vi "Tag Watchlist Example.vi"() -> ()   [LabVIEW 2020]
uses:
  Tag/Tag.lvclass/Tag.ctl
  e068aabd-e1ea-42e0-beff-873828abce71.vi
  d3806a0d-e09d-4e85-9d5e-98b09324ad8a.vi
  Tag/Construct.vi
  Core/Write Tag Value_ByRef.vi
  Tag/Write Value with Timestamp.vi
  Tag/Set Properties from Initial.vi
  Core/Add Tag.vi
  Tag/Tag.lvclass
  Core/Tag Core.lvclass
  Watchlist/Tag Watchlist.lvlib
  26ea3595-a312-4975-b521-b090e0f49d92.vi
panel:
  in  "Launch Watchlist":bool
  in  "stop":bool
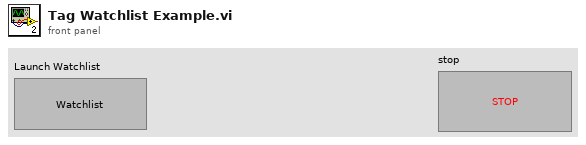
[diagram p1: front panel]
types:
  T1 = cluster{"Name":string, "Value":dbl, "Enable":bool}
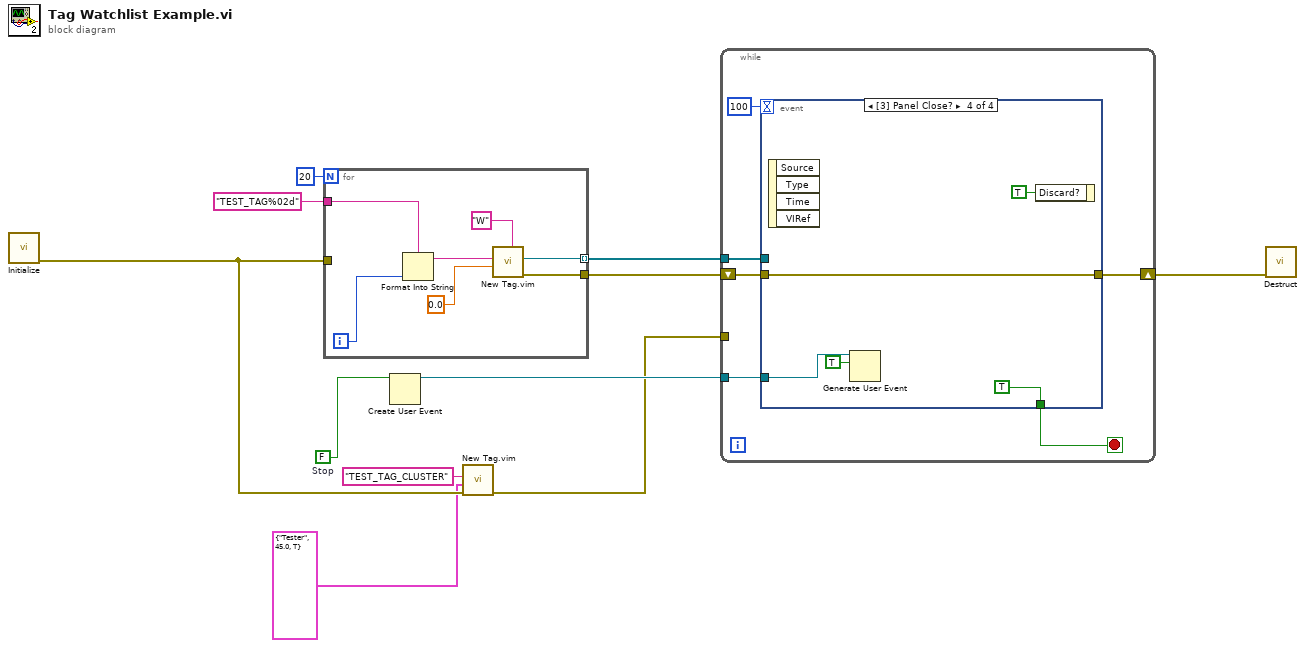
[diagram p0: block diagram]
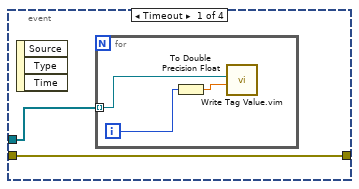
[diagram p2: hidden frame]
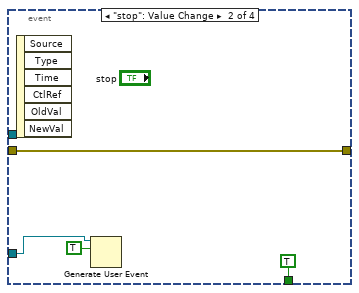
[diagram p3: hidden frame]
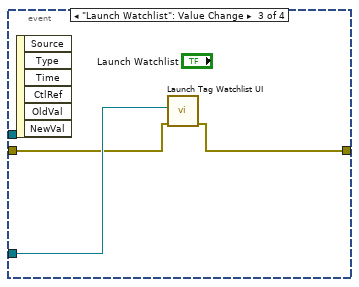
[diagram p4: hidden frame]
diagram:
  w7 = FALSE  # Stop
  n1 = call "Initialize.vi"() -> ("error out"=w4:errorcluster)  [unwired: 11 in]
  n2 = for {
    N: 20 -> [_]
    tunnel: "TEST_TAG%02d" -> [w18]
    tunnel: [w14] -> w9
    tunnel: [w13] -> w5 mode=indexing
    tunnel: w4 -> [_]
    i -> [w17]
    n3 = Format Into String(format string=w18, w17) -> (resulting string=w16:string)  [unwired: 2 in, 1 out]
    n4 = call "New Tag.vim"("Units (none)"="W", "Initial Value"=0.0, "Tag Name"=w16) -> ("error out"=w14:errorcluster, "Tag Ref out"=w13:refnum<data-value>)  [unwired: 7 in]
  }
  n5 = Create User Event(user event datatype=w7) -> (user event=w6:refnum<user-event>)  [unwired: 1 in, 1 out]
  n6 = call "New Tag.vim"("error in (no error)"=w4, "Initial Value"=T1 {"Name"="Tester", "Value"=45.0, "Enable"=TRUE}, "Tag Name"="TEST_TAG_CLUSTER") -> ("error out"=w1:errorcluster)  [unwired: 7 in, 1 out]
  n7 = while {
    shift-right: [w22] -> w8
    shift-left: w9 -> [w23]
    tunnel: w6 -> [w21]
    tunnel: w5 -> [w19]
    tunnel: w1 -> [_]
    stop <- w24 stop-if-true
    n8 = event shown="[3] Panel Close?" {
      selector: _ -> [_ _ _ _]
      dyn-events: _ -> [_ _ _ _]
      timeout: 100 -> [_ _ _ _]
      tunnel: [_ TRUE _ TRUE] -> w24
      tunnel: w23 -> [w26 w33 w35 w39]
      tunnel: [w26 w33 w34 w39] -> w22
      tunnel: w21 -> [_ w30 w36 w38]
      tunnel: w19 -> [w25 _ _ _]
      event Timeout {
        n9 = event-data() -> ()  [unwired: 1 in, 3 out]
        n10 = for {
          tunnel: w25 -> [w29] mode=indexing
          i -> [w28]
          n11 = To Double Precision Float(number=w28) -> (double precision float=w27:dbl)
          n12 = call "Write Tag Value.vim"("Value"=w27, "Tag Name(s)/Ref(s)"=w29) -> ()  [unwired: 8 in, 2 out]
        }
      }
      event "stop": Value Change {
        n13 = event-data() -> ()  [unwired: 1 in, 6 out]
        n14 = Generate User Event(user event=w30, event data cluster=TRUE ("event data")) -> ()  [unwired: 2 in, 2 out]
      }
      event "Launch Watchlist": Value Change {
        n15 = event-data() -> ()  [unwired: 1 in, 6 out]
        n16 = call "Launch Tag Watchlist UI.vi"("error in (no error)"=w35, "Shutdown Event"=w36) -> ("error out"=w34:errorcluster)  [unwired: 9 in]
      }
      event Panel Close? {
        n17 = event-data() -> ()  [unwired: 1 in, 4 out]
        n18 = Generate User Event(user event=w38, event data cluster=TRUE ("event data")) -> ()  [unwired: 2 in, 2 out]
        n19 = event-data("Discard?"=TRUE) -> ()  [unwired: 1 in, 1 out]
      }
    }
  }
  n20 = call "Destruct.vi"("error in (no error)"=w8) -> ()  [unwired: 10 in, 1 out]
